vi "MS Initialization.vi"(6 "PID Cluster":T2={"L1 to L4 PID Cluster"={"L1 PID Gains"={"Kp"=0.005, "Kd"=0.5, "Ki"=0.0005}, "L2 PID Gains"={"Kp"=0.01, "Kd"=1.0, "Ki"=0.005}, "L3 PID Gains"={"Kp"=0.05, "Kd"=1.0, "Ki"=0.0005}, "L4 PID Gains"={"Kp"=0.1, "Kd"=0.1, "Ki"=0.0005}}, "Stage PID Cluster"={"Stage Z PID"={"Kp"=0.0005, "Kd"=0.001, "Ki"=0.0}, "Stage Y PID"={"Kp"=0.0003, "Kd"=0.01, "Ki"=0.0}, "Stage X PID"={"Kp"=0.0003, "Kd"=0.01, "Ki"=0.0}}, "OCT Z PID Gains"={"Kp"=0.0003, "Kd"=0.0001, "Ki"=0.01}}, 8 "error in":errorcluster, 9 "Offset Home 2 RCM":dbl[](array[numeric])=[0.0, 0.0, 0.0, 0.0], 10 "Prev Posit Cluster":T3={"Prev L1 to L4 Posit"=[0.0, 0.0, 0.0, 0.0], "Prev Stage Posit"=[6.0, 6.0, 6.0], "Prev OCT Z Posit"=0.0}, 11 "FPGA VI Reference In":refnum<k20>) -> (0 "error out":errorcluster, 2 "Last Posit Cluster":T1={"Last L1 to L4 Posit"=[0.0, 0.0, 0.0, 0.0], "Last Stage Posit"=[6.0, 6.0, 6.0], "Last OCT Z Posit"=0.0}, 3 "FPGA VI Reference Out":refnum<k20>)   [LabVIEW 2016]
uses:
  <vilib>/Platform/TimedLoop/XDataNode/timing_clust.ctl
  <vilib>/Platform/TimedLoop/XDataNode/nitl_modes.ctl
  <vilib>/Platform/TimedLoop/XDataNode/wakeup.ctl
  Global Variables.vi
  <vilib>/platform/TimedLoop/XDataNode/XDataNode.xnode
  <vilib>/Platform/TimedLoop/XDataNode/XDNodeRunTimeDep.lvlib
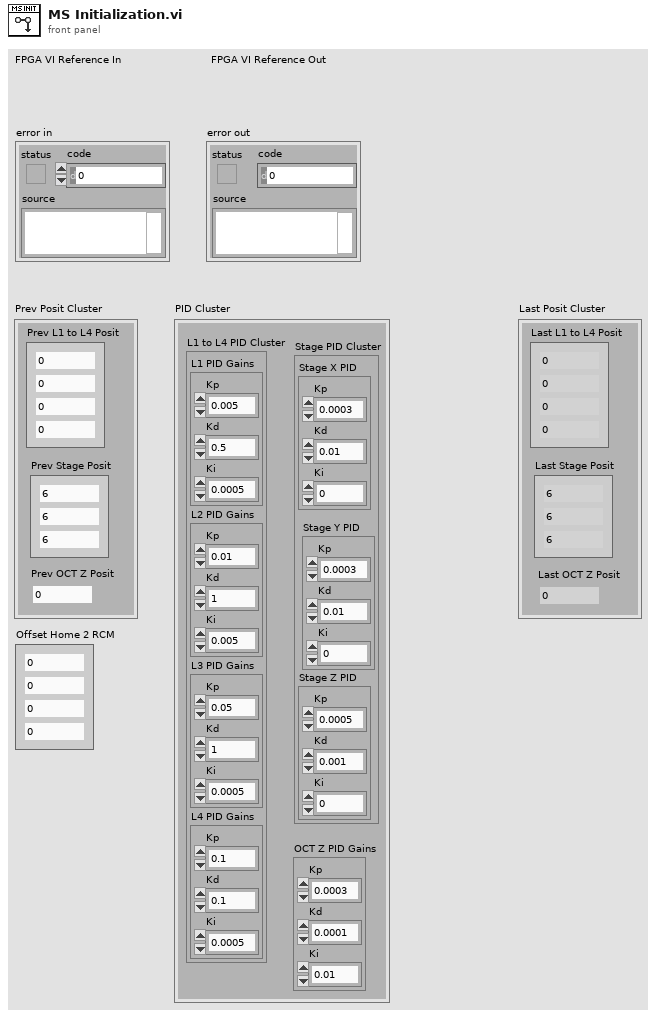
[diagram p1: front panel]
types:
  T1 = cluster{"Last L1 to L4 Posit":dbl[], "Last Stage Posit":dbl[], "Last OCT Z Posit":dbl}
  T2 = cluster{"L1 to L4 PID Cluster":cluster{"L1 PID Gains":cluster{"Kp":dbl, "Kd":dbl, "Ki":dbl}, "L2 PID Gains":cluster{"Kp":dbl, "Kd":dbl, "Ki":dbl}, "L3 PID Gains":cluster{"Kp":dbl, "Kd":dbl, "Ki":dbl}, "L4 PID Gains":cluster{"Kp":dbl, "Kd":dbl, "Ki":dbl}}, "Stage PID Cluster":cluster{"Stage Z PID":cluster{"Kp":dbl, "Kd":dbl, "Ki":dbl}, "Stage Y PID":cluster{"Kp":dbl, "Kd":dbl, "Ki":dbl}, "Stage X PID":cluster{"Kp":dbl, "Kd":dbl, "Ki":dbl}}, "OCT Z PID Gains":cluster{"Kp":dbl, "Kd":dbl, "Ki":dbl}}
  T3 = cluster{"Prev L1 to L4 Posit":dbl[], "Prev Stage Posit":dbl[], "Prev OCT Z Posit":dbl}
  T4 = cluster{"Stop Vacuum":bool, "Vacuum Force":i8, "Max Limit [mmHg]":dbl, "Slide in":i8, "Irrigation?":bool}
  T5 = typedef "XDNodeRunTimeDep.lvlib/timing_clust.ctl" = cluster{"Expected End [f-1]":u64, "Actual End [f-1]":u64, "Finished Late? [f-1]":bool, "Expected End [i-1]":u64, "Actual End [i-1]":u64, "Finished Late? [i-1]":bool, "Expected Start [i]":u64, "Actual Start [i]":u64, "Expected Start [f]":u64, "Actual Start [f]":u64, "Source Name":string, "Structure Name":string, "Period":i64, "Deadline":i64, "Offset":i64, "Start":i64, "Priority":i32, "Timeout":i32, "Mode":T6, "Wakeup Reason":T7, "Error":errorcluster, "Source Type":string, "Secondary Source Type":string, "Global End Time":u64, "Global Start Time":u64, "Frame Duration":u64, "Iteration Duration":u64, "Assigned CPU":i32, "I/O Scan Engine Mode":u32}
  T6 = typedef "XDNodeRunTimeDep.lvlib/nitl_modes.ctl" = enum32{"No Change", "Process missed periods, maintain original phase", "Discard missed periods, maintain original phase", "Process missed periods, ignore original phase", "Discard missed periods, ignore original phase"}
  T7 = typedef "XDNodeRunTimeDep.lvlib/wakeup.ctl" = enum32{"Normal", "Aborted", "Asynchronous wakeup", "Timing source error", "Timed loop error", "Timeout"}
  T8 = cluster{"L1 PID Gains":cluster{"Kp":dbl, "Kd":dbl, "Ki":dbl}, "L2 PID Gains":cluster{"Kp":dbl, "Kd":dbl, "Ki":dbl}, "L3 PID Gains":cluster{"Kp":dbl, "Kd":dbl, "Ki":dbl}, "L4 PID Gains":cluster{"Kp":dbl, "Kd":dbl, "Ki":dbl}}
  T9 = cluster{"Stage Z PID":cluster{"Kp":dbl, "Kd":dbl, "Ki":dbl}, "Stage Y PID":cluster{"Kp":dbl, "Kd":dbl, "Ki":dbl}, "Stage X PID":cluster{"Kp":dbl, "Kd":dbl, "Ki":dbl}}
  T10 = cluster{"Accurus button":bool[], "Accurus engaged?":bool, "Vacuum Force":i32, "Accurus Ch. A Vout":dbl, "Accurus Ch. B Vout":dbl, "Irrigation engaged?":bool}
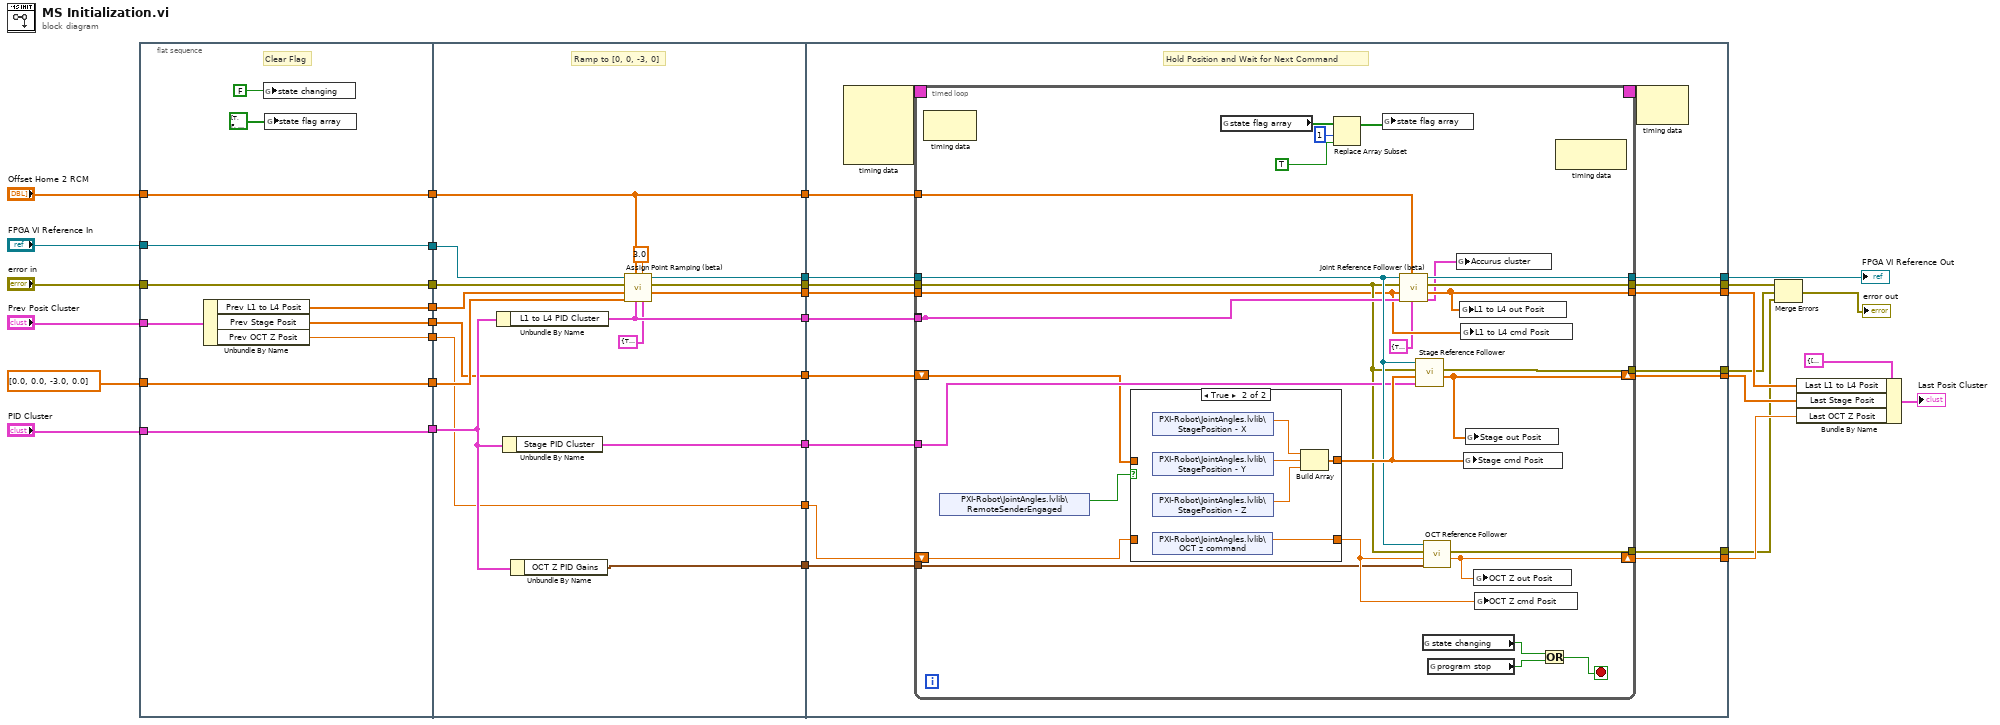
[diagram p0: block diagram]
diagram:
  n1 = flat-sequence {
    tunnel: "Prev Posit Cluster" -> [w42]
    tunnel: dbl[] [0.0, 0.0, -3.0, 0.0] ("First Trk Pt 2") -> [w41]
    tunnel: [w41] -> w31
    tunnel: [w40] -> w30
    tunnel: [w39] -> w29
    tunnel: "PID Cluster" -> [w39]
    tunnel: "error in" -> [w38]
    tunnel: [w38] -> w26
    tunnel: "Offset Home 2 RCM" -> [w37]
    tunnel: [w37] -> w24
    tunnel: [w36] -> w23
    tunnel: "FPGA VI Reference In" -> [w36]
    tunnel: [w35] -> w4
    tunnel: [w34] -> w2
    tunnel: w31 -> [w59]
    tunnel: w30 -> [w60]
    tunnel: w29 -> [w55]
    tunnel: w26 -> [w58]
    tunnel: w24 -> [w48]
    tunnel: w23 -> [w57]
    tunnel: [w54] -> w21
    tunnel: [w53] -> w20
    tunnel: [w52] -> w19
    tunnel: [w51] -> w18
    tunnel: [w50] -> w17
    tunnel: [w49] -> w16
    tunnel: [w48] -> w15
    tunnel: w4 -> [w47]
    tunnel: [w47] -> w3
    tunnel: w2 -> [w46]
    tunnel: [w46] -> w1
    tunnel: w21 -> [w76]
    tunnel: w20 -> [w75]
    tunnel: w19 -> [w74]
    tunnel: w18 -> [w73]
    tunnel: w17 -> [w72]
    tunnel: w16 -> [w71]
    tunnel: w15 -> [w70]
    tunnel: [w69] -> w14
    tunnel: [w68] -> w8
    tunnel: [w67] -> w11
    tunnel: [w66] -> w10
    tunnel: [w65] -> w9
    tunnel: [w64] -> w6
    tunnel: [w63] -> w5
    tunnel: w3 -> [w62]
    tunnel: w1 -> [w61]
    frame #0 {
      # "Clear Flag"
      n2 = Unbundle By Name(w42) -> ("Prev L1 to L4 Posit"=w40:dbl[], "Prev Stage Posit"=w35:dbl[], "Prev OCT Z Posit"=w34:dbl)
      n3 = global write "Global Variables.vi" "state changing"(FALSE ("state changing")) -> ()
      n4 = global write "Global Variables.vi" "state flag array"(bool[] [TRUE, FALSE, FALSE, FALSE, FALSE, FALSE, FALSE, FALSE, FALSE] ("state flag array")) -> ()
    }
    frame #1 {
      # "Ramp to [0, 0, -3, 0]"
      n5 = Unbundle By Name(w55) -> ("L1 to L4 PID Cluster"=w52:T8)
      n6 = Unbundle By Name(w55) -> ("Stage PID Cluster"=w51:T9)
      n7 = Unbundle By Name(w55) -> ("OCT Z PID Gains"=w50:cluster{"Kp":dbl, "Kd":dbl, "Ki":dbl})
      n8 = call "Assign Point Ramping (beta).vi"("Accurus Ctrl Cluster"=T4 {"Stop Vacuum"=TRUE, "Vacuum Force"=0, "Max Limit [mmHg]"=600.0, "Slide in"=0, "Irrigation?"=FALSE}, "Ramp Time [sec]"=3.0, "L1 to L4 PID Cluster"=w52, "Offset Home2RCM"=w48, "Destination Posit Array [mm]"=w59, "Previous Posit Array"=w60, "error in"=w58, "FPGA VI Reference In"=w57) -> ("Last L1 to L4 Posit"=w49:dbl[], "error out"=w53:errorcluster, "FPGA VI Reference Out"=w54:refnum<k20>)  [unwired: 1 in]
    }
    frame #2 {
      # "Hold Position and Wait for Next Command"
      n9 = node-c288() -> (w78:T5)  [unwired: 4 in]
      n10 = timed-loop {
        timing: w78 -> [_]
        timing-out: [_] -> w77
        tunnel: w76 -> [w97]
        tunnel: w75 -> [w93]
        tunnel: [w96] -> _
        tunnel: w74 -> [w96]
        tunnel: w73 -> [w95]
        tunnel: w72 -> [w94]
        tunnel: w71 -> [w92]
        tunnel: w70 -> [w91]
        tunnel: [w90] -> w69
        tunnel: [w89] -> w68
        tunnel: [w88] -> w67
        tunnel: [w85] -> w64
        tunnel: [w84] -> w63
        shift-right: [w87] -> w66
        shift-left: w62 -> [w82]
        shift-right: [w86] -> w65
        shift-left: w61 -> [w81]
        stop <- w106 stop-if-true
        n11 = node-c288() -> ()  [unwired: 1 in, 1 out]
        n12 = shared-variable "PXI-Robot\\JointAngles.lvlib\\RemoteSenderEngaged"() -> (w83:bool)  [unwired: 1 in, 1 out]
        n13 = case shown="True" w83 {
          tunnel: [w107 w113] -> w99
          tunnel: [w108 w112] -> w98
          tunnel: w82 -> [w108 _]
          tunnel: w81 -> [w107 _]
          frame False {
          }
          frame True {
            n14 = shared-variable "PXI-Robot\\JointAngles.lvlib\\StagePosition - X"() -> (w109:dbl)  [unwired: 1 in, 1 out]
            n15 = shared-variable "PXI-Robot\\JointAngles.lvlib\\StagePosition - Y"() -> (w110:dbl)  [unwired: 1 in, 1 out]
            n16 = shared-variable "PXI-Robot\\JointAngles.lvlib\\StagePosition - Z"() -> (w111:dbl)  [unwired: 1 in, 1 out]
            n17 = shared-variable "PXI-Robot\\JointAngles.lvlib\\OCT z command"() -> (w113:dbl)  [unwired: 1 in, 1 out]
            n18 = Build Array(w109, w110, w111) -> (w112:dbl[])
          }
        }
        n19 = global read "Global Variables.vi" "state flag array"() -> (w103:bool[])
        n20 = Replace Array Subset(array=w103, new element=TRUE ("new element/subarray"), index=1) -> (w102:bool[])
        n21 = global write "Global Variables.vi" "state flag array"(w102) -> ()
        n22 = call "Joint Reference Follower (beta).vi"("Accurus Ctrl Cluster"=T4 {"Stop Vacuum"=TRUE, "Vacuum Force"=0, "Max Limit [mmHg]"=600.0, "Slide in"=0, "Irrigation?"=FALSE}, "Offset Home2RCM [deg/mm]"=w91, "PID Ctrl Cluster"=w96, "Ref Array [deg/mm]"=w92, "error in"=w93, "FPGA VI Reference In"=w97) -> ("Accurus Output Cluster"=w79:T10, "Output Posit Array [deg/mm]"=w88:dbl[], "error out"=w89:errorcluster, "FPGA VI Reference Out"=w90:refnum<k20>)  [unwired: 2 in]
        n23 = call "Stage Reference Follower.vi"("Stage PID Cluster"=w95, "Stage cmd Posit [mm]"=w98, "error in"=w93, "FPGA VI Reference In"=w97) -> ("Stage out Posit [mm]"=w87:dbl[], "error out"=w85:errorcluster)  [unwired: 5 in, 1 out]
        n24 = global read "Global Variables.vi" "state changing"() -> (w105:bool)
        n25 = call "OCT Reference Follower.vi"("OCT Z PID Gains"=w94, "OCT  Z cmd Posit [mm]"=w99, "error in"=w93, "FPGA VI Reference In"=w97) -> ("OCT  Z out Posit [mm]"=w86:dbl, "error out"=w84:errorcluster)  [unwired: 5 in, 1 out]
        n26 = global read "Global Variables.vi" "program stop"() -> (w104:bool)
        n27 = global write "Global Variables.vi" "Accurus cluster"(w79) -> ()
        n28 = global write "Global Variables.vi" "L1 to L4 out Posit"(w88) -> ()
        n29 = global write "Global Variables.vi" "L1 to L4 cmd Posit"(w92) -> ()
        n30 = global write "Global Variables.vi" "Stage cmd Posit"(w98) -> ()
        n31 = global write "Global Variables.vi" "Stage out Posit"(w87) -> ()
        n32 = global write "Global Variables.vi" "OCT Z out Posit"(w86) -> ()
        n33 = global write "Global Variables.vi" "OCT Z cmd Posit"(w99) -> ()
        n34 = Or(x=w105, y=w104) -> (x .or. y?=w106:bool)
        n35 = node-c288() -> ()  [unwired: 1 in, 1 out]
      }
      n36 = node-c288(w77) -> ()  [unwired: 1 out]
    }
  }
  n37 = Merge Errors(w8, w6, w5) -> (→"error out":errorcluster)
  n38 = Bundle By Name(cluster=T1 {"Last L1 to L4 Posit"=[0.0, 0.0, 0.0, 0.0], "Last Stage Posit"=[6.0, 6.0, 6.0], "Last OCT Z Posit"=0.0} ("Last Posit Cluster 2"), "Last L1 to L4 Posit"=w11, "Last Stage Posit"=w10, "Last OCT Z Posit"=w9) -> (→"Last Posit Cluster":T1)
  "FPGA VI Reference Out" <- w14
